vi "FeedForSensor.vi"() -> ()   [LabVIEW 2020]
uses:
  Framework/Robot Global Data.vi
panel:
  in  "NoWait":bool
  in  "LowerSpeed":dbl
  in  "UpperSpeed":dbl
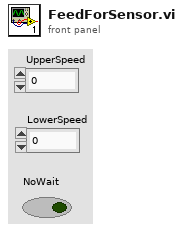
[diagram p1: front panel]
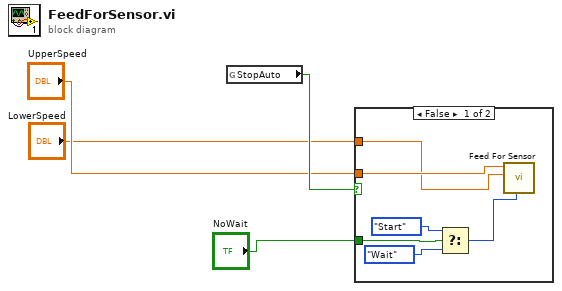
[diagram p0: block diagram]
diagram:
  n1 = global read "Robot Global Data.vi" "StopAuto"() -> (w4:bool)
  n2 = case shown="False" w4 {
    tunnel: "NoWait" -> [w8 _]
    tunnel: "UpperSpeed" -> [w7 _]
    tunnel: "LowerSpeed" -> [w6 _]
    frame False {
      n3 = Select(t=enum16{"Start", "Wait"}."Start" ("Synchronization"), s=w8, f=enum16{"Start", "Wait"}."Wait" ("Synchronization")) -> (s? t:f=w5:enum16{"Start", "Wait"})
      n4 = call "Feed For Sensor.vi"("Synchronization"=w5, "Lower"=w6, "Upper"=w7) -> ()  [unwired: 8 in, 1 out]
    }
    frame True {
    }
  }
